vi "MarvinReport.vi"(0 "HEADER1":string="===================================================================\r\n||  Functional and Performance Test  For  DUAL-SERVO- L O W E R  ||\r\n||  P/N  TLM132XX501    S/N:001    Power-Input:18,28,32 +/-0.5V  ||\r\n||  Date:6/12/2007    Time: 15-00  Test-Conductor: Itzik         ||\r\n||  Tester P/N yyyy-yyyyyy-yyyy    S/N:01                        ||\r\n||  POWER SUPPLY P/N xxxxx                                       ||\r\n||  Remarks:                                                     ||\r\n||  You can write here what ever you want                        ||\r\n||                                                               ||\r\n===================================================================", 1 "ATR Or":refnum<vi>, 2 "Steps   pfull":string[][](table)=array602x15[9030 elements] caption="ATR", 3 "Footer UUT":string, 5 "pageNum":i32=13, 6 "InputHeaderArray":string[][](array[string]), 7 "FILE NAME":string="d", 9 "Report Folder":path=path "C:/EPD/ATRS", 11 "Open File":bool caption="Open", 12 "error in (no error)":errorcluster, 13 "REV":string, 14 "Test-Conductor":string) -> (4 "path out":path, 15 "error out":errorcluster)   [LabVIEW 2017]
uses:
  <vilib>/Utility/miscctls.llb/LVRowAndColumnUnsignedTypeDef.ctl
  <vilib>/Utility/NIReport.llb/Append Image to Report (path wrap).vi
  <vilib>/Utility/NIReport.llb/Append Text Table to Report (wrap).vi
  <vilib>/Utility/NIReport.llb/Append Report Text (str wrap).vi
  <vilib>/Utility/NIReport.llb/NI_report.lvclass
  <vilib>/Utility/NIReport.llb/Word/NI_Word.lvclass
  <vilib>/addons/_office/NI_ReportGenerationToolkit.lvlib
panel:
  out "Steps   p31":string[][](table)=[["6.1", "Visual Inspection", "", "", "", "", ""], ["6.1.1", "Verification of Components Not Installed", "N/A", "-", "", "", ""], ["", "", "", "", "", "", ""], ["6.1.2", "Manufacturing Defects", "N/A", "-", "", "", ""], ["", "", "", "", "", "", ""], ["6.2", "Power Supply Testing", "", "", "", "", ""], ["6.2.1", "Input Current Drawn", "", "", "", "", ""], ["6.2.1.1", "DC Input Current", "< 150", "-", "mA", "", ""], ["", "", "", "", "", "", ""], ["6.2.2", "Power Supply Voltages", "", "", "", "", ""], ["6.2.2.1", "12V", "12.0", "+/-0.500", "V", "", ""], ["6.2.2.2", "5V", "5.0", "+/-0.200", "V", "", ""], ["6.2.2.3", "3.3V", "3.3", "+/-0.100", "V", "", ""], ["6.2.2.4", "1.8V", "1.8", "+/-0.100", "V", "", ""], ["", "", "", "", "", "", ""], ["7", "Functional Test Procedure", "", "", "", "", ""], ["7.1", "Weight Check", "4180", "+/-10.00", "gr", "", ""], ["", "", "", "", "", "", ""], ["7.2", "Insulation Resistance Test", "", "", "", "", ""], ["7.2.1", "J3.B to Chassis", "> 1M", "-", "ohms", "", ""], ["7.2.2", "J1.16 to Chassis", "> 100K", "-", "ohms", "", ""], ["", "", "", "", "", "", ""], ["7.2", "Bonding Resistance", "", "", "", "", ""], ["7.2.3", "J1 Body to Chassis", "< 2m", "-", "ohms", "", ""], ["7.2.4", "J2  Body to Chassis", "< 2m", "-", "ohms", "", ""], ["7.2.5", "J3  Body to Chassis", "< 2m", "-", "ohms", "", ""], ["", "", "", "", "", "", ""], ["7.2.1", "CANbus Resistance Test", "", "", "", "", ""], ["7.2.1.1", "J1.17 to J1.18", "> 10K", "-", "ohms", "", ""], ["", "", "", "", "", "", ""], ["7.3", "Sealing Test", "N/A", "-", "", "", ""], ["", "", "", "", "", "", ""], ["7.4", "Communication Test", "", "", "", "", ""], ["7.4.1", "Serial RS-232", "N/A", "-", "", "", ""], ["7.4.2", "CAN Bus", "N/A", "-", "", "", ""], ["", "", "", "", "", "", ""], ["7.5", "Performances Tests", "", "", "", "", ""], ["7.5.1", "Reverse Polarity Test", "", "", "", "", ""], ["7.5.1.1", "DC Input Current", "< 1", "-", "mA", "", ""], ["", "", "", "", "", "", ""], ["7.5.2", "Enable Test", "", "", "", "", ""], ["7.5.2.1", "Fan Speed before Opened Enable ", "6000", "+/-200.0", "rpm", "", ""], ["7.5.2.2", "Fan Speed at Opened Enable ", "0", "+/-200.0", "rpm", "", ""], ["7.5.2.3", "Fan Speed at Closed Enable ", "6000", "+/-200.0", "rpm", "", ""], ["7.5.2.4", "Motor Rotation Direction", "Counter-clockwise (Inlet)", "-", "", "", ""], ["", "", "", "", "", "", ""], ["7.5.3", "Stop Time Test ", "", "", "", "", ""], ["7.5.3.1", "Motor Stop time", "< 50", "-", "sec", "", ""], ["", "", "", "", "", "", ""], ["7.5.4", "Speed Command Test", "", "", "", "", ""], ["7.5.4.1", "Fan Speed", "6000", "+/-200.0", "rpm", "", ""], ["7.5.4.2", "Fan Speed", "11500", "+/-200.0", "rpm", "", ""], ["7.5.4.3", "Fan Speed", "15100", "+/-200.0", "rpm", "", ""], ["", "", "", "", "", "", ""], ["7.5.5", "Temperature Sensor Calibration Test", "", "", "", "", ""], ["7.5.5.1", "Sensor Reading Analog Offset", "0", "+/-0.100", ".", "", ""], ["", "", "", "", "", "", ""], ["7.5.6", "Temperature Control Algorithm Test", "", "", "", "", ""], ["7.5.6.1", "Tair <   68 ± 2 oC", "6000", "+/-200.0", "rpm", "", ""], ["7.5.6.2", "Measured Temp.", "", "", "Deg.", "", ""], ["7.5.6.3", "Tair >= 68 ± 2 oC", "11500", "+/-200.0", "rpm", "", ""], ["7.5.6.4", "Transition Temp.", "", "", "Deg.", "", ""], ["7.5.6.5", "Tair >= 88 ± 2 oC", "15100", "+/-400.0", "rpm", "", ""], ["7.5.6.6", "Transition Temp.", "", "", "Deg.", "", ""], ["7.5.6.7", "Tair <= 80 ± 2 oC", "11500", "+/-200.0", "rpm", "", ""], ["7.5.6.8", "Transition Temp.", "", "", "Deg.", "", ""], ["7.5.6.9", "Tair <= 60 ± 2 oC", "6000", "+/-200.0", "rpm", "", ""], ["7.5.6.10", "Transition Temp.", "", "", "Deg.", "", ""], ["", "", "", "", "", "", ""], ["7.5.7", "Burn-in Test", "", "", "", "", ""], ["7.5.7.1", "DC Input Current", "50", "+/-7.000", "A", "", ""], ["7.5.7.2", "Fan Speed", "15100", "+/-400.0", "rpm", "", ""], ["7.5.7.3", "Ambient Temperature", "25", "+/-13.00", "Deg.", "", ""], ["7.5.7.4", "After 10 min of operation", "", "-", "Deg.", "", ""], ["7.5.7.5", "After 20 min of operation", "", "-", "Deg.", "", ""], ["7.5.7.6", "After 30 min of operation", "", "-", "Deg.", "", ""], ["", "", "", "", "", "", ""], ["8", "Auxiliary", "", "", "", "", ""], ["8.1", "Auxiliary Cooling Fan ON", "60", "+/-2.00", "Deg.", "", ""], ["8.2", "Fan status", "ON", "-", "-", "", ""], ["8.3", "Auxiliary Cooling Fan OFF", "55", "+/-2.00", "Deg.", "", ""], ["8.4", "Fan status", "OFF", "-", "-", "", ""], ["", "", "", "", "", "", ""], ["9", "Motor Temp. Test", "", "", "", "", ""], ["9.1", "60 Degree", "60", "+/-2.00", "Deg.", "", ""], ["9.2", "90 Degree", "90", "+/-2.00", "Deg.", "", ""], ["9.3", "110 Degree", "110", "+/-2.00", "Deg.", "", ""]] caption="ATR"
  out "error out 2":errorcluster
  out "RefArr":u32[](array[numeric])
  in  "Tab Control":T1(tab)=enum."Headers and more"
  out "ERRORS\nLIST":string="<pre>Summery of Results (Fails Only) :   Pos.Cmnd.=0.5V F.B. - FAIL !\t   \nPos.Cmnd.=2.0V F.B. - FAIL !\t       Pos.Cmnd.=4.5V F.B. - FAIL !\t  \nPos.Cmnd.=0.5V F.B  - FAIL !\t       Pos.Cmnd.=2.0V F.B. - FAIL !\t\nPos.Cmnd.=4.5V F.B. - FAIL !\t       Pot. / Pos.Cmnd. 1.5v - FAIL !\t   \nPot./Pos.Cmnd.2.0v  - FAIL !\t       Pot. / Pos.Cmnd. 3.5v - FAIL !\t   \nRelay-->RESET  - FAIL !\t            Relay --> SET - FAIL !\t</pre>"
  out "Steps   p1":string[][](table)=[["Load Firmware - reset", "-", "-", "-", "-", ""], ["Test Communication", "-", "-", "-", "-", ""], ["Set S/N", "-", "-", "-", "-", ""], ["Set Board Number", "-", "-", "-", "-", ""], [" ", "", "", "", "", ""], ["Test Communication", "-", "-", "-", "-", ""], ["Get S/N", "-", "-", "-", "", ""], ["Get Board Number", "-", "-", "-", "", ""], ["Get FW", "-", "-", "-", "", ""], ["Small position command", "", "", "", "", ""], ["Measure delta", "", "", "", "", ""], ["Velocity command", "", "", "", "", ""], ["Velocity command", "", "", "", "", ""], ["Velocity command", "", "", "", "", ""], ["Velocity command", "", "", "", "", ""], ["Velocity command", "", "", "", "", ""]] caption="ATR"
  out "Steps   p2":string[][](table)=[["Load Firmware - reset", "-", "-", "-", "-", ""], ["Test Communication", "-", "-", "-", "-", ""], ["Set S/N", "-", "-", "-", "-", ""], ["Set Board Number", "-", "-", "-", "-", ""], [" ", "", "", "", "", ""], ["Test Communication", "-", "-", "-", "-", ""], ["Get S/N", "-", "-", "-", "", ""], ["Get Board Number", "-", "-", "-", "", ""], ["Get FW", "-", "-", "-", "", ""], ["Small position command", "", "", "", "", ""], ["Measure delta", "", "", "", "", ""], ["Velocity command", "", "", "", "", ""], ["Velocity command", "", "", "", "", ""], ["Velocity command", "", "", "", "", ""], ["Velocity command", "", "", "", "", ""], ["Velocity command", "", "", "", "", ""]] caption="ATR"
  out "Steps   p3":string[][](table)=[["Load Firmware - reset", "-", "-", "-", "-", ""], ["Test Communication", "-", "-", "-", "-", ""], ["Set S/N", "-", "-", "-", "-", ""], ["Set Board Number", "-", "-", "-", "-", ""], [" ", "", "", "", "", ""], ["Test Communication", "-", "-", "-", "-", ""], ["Get S/N", "-", "-", "-", "", ""], ["Get Board Number", "-", "-", "-", "", ""], ["Get FW", "-", "-", "-", "", ""], ["Small position command", "", "", "", "", ""], ["Measure delta", "", "", "", "", ""], ["Velocity command", "", "", "", "", ""], ["Velocity command", "", "", "", "", ""], ["Velocity command", "", "", "", "", ""], ["Velocity command", "", "", "", "", ""], ["Velocity command", "", "", "", "", ""]] caption="ATR"
  in  "Fail  Button":bool
  in  "Pass  Button":bool
  # "e"
  # "e"
  # "<pre>"
  # "for html"
  # "for html"
  # "</pre>"
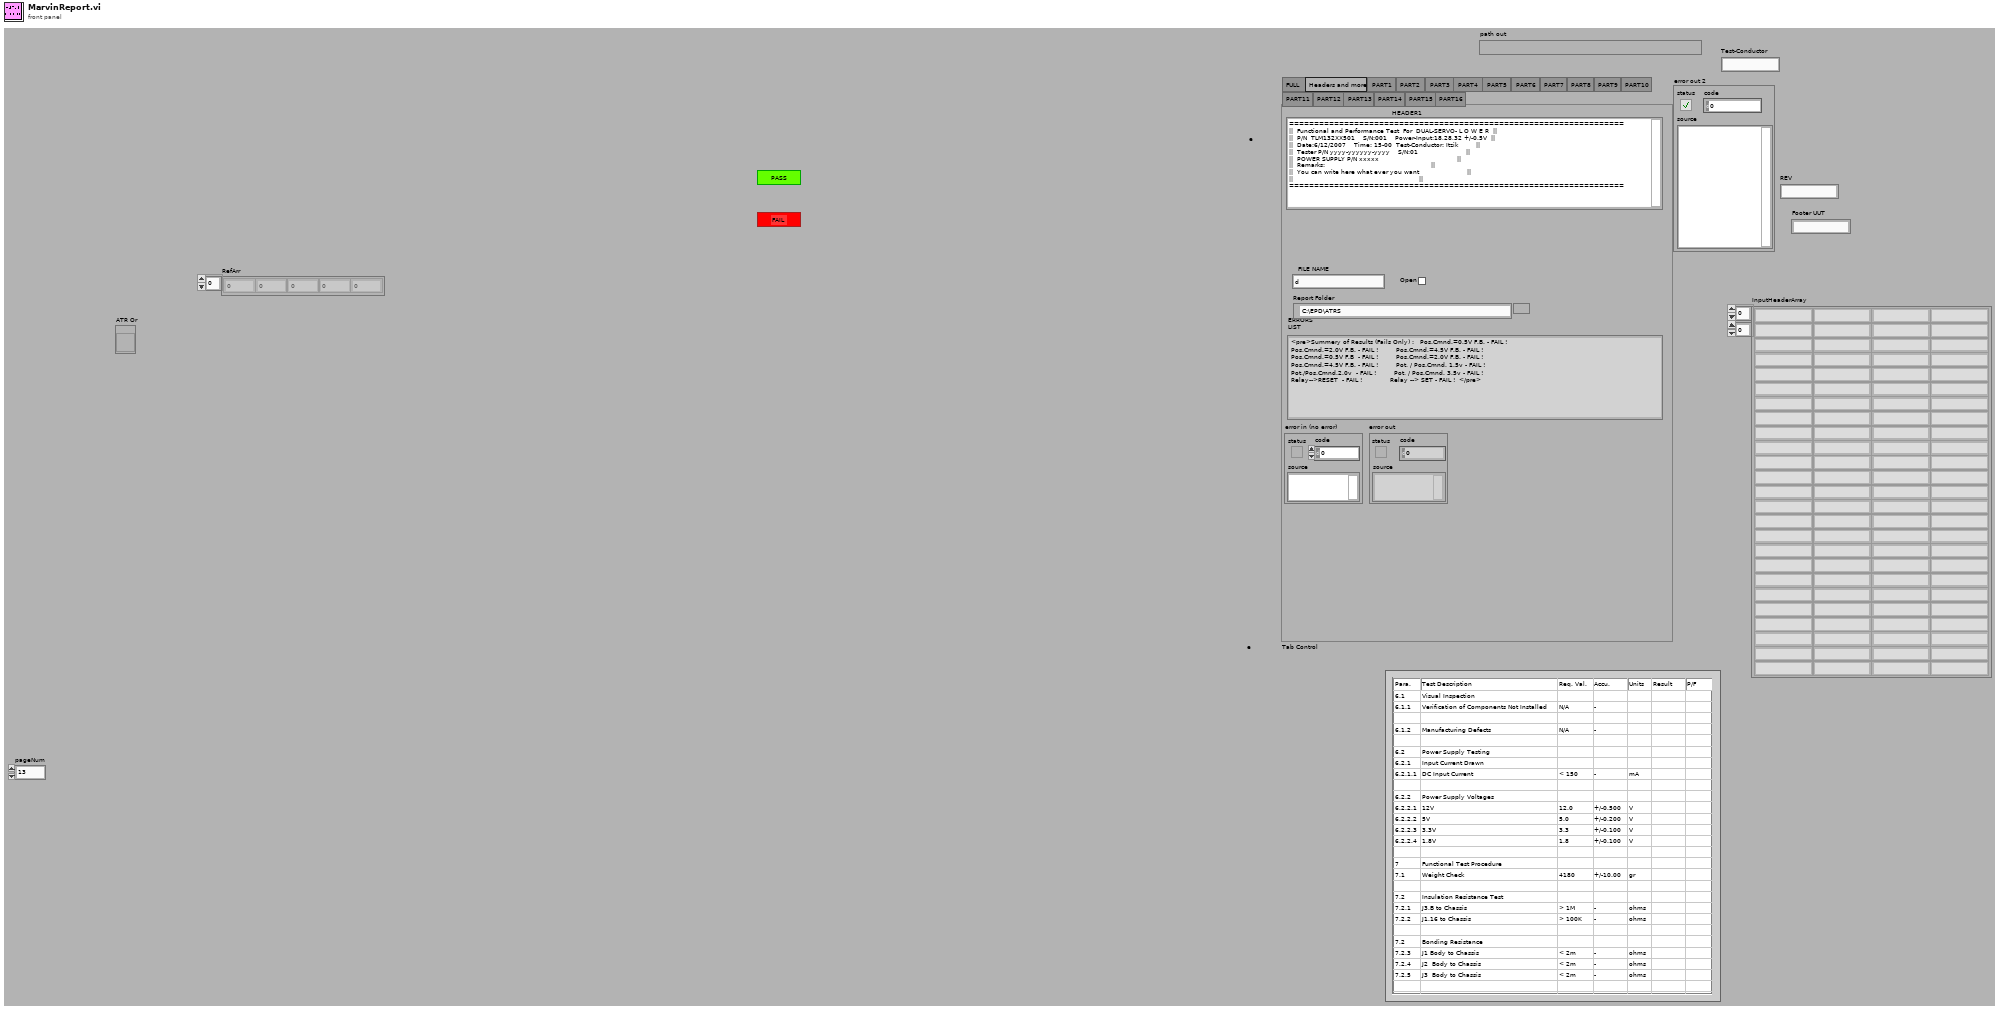
[diagram p1: front panel]
types:
  T1 = enum32{"FULL", "Headers and more", "PART1 ", "PART2 ", "PART3 ", "PART4 ", "PART5 ", "PART6 ", "PART7", "PART8", "PART9", "PART10", "PART11", "PART12", "PART13", "PART14", "PART15", "PART16"}
  T2 = typedef "LVRowAndColumnUnsignedTypeDef.ctl" = cluster{"Row":u32, "Column":u32}
  T3 = cluster{"position (excel)":cluster{"row":i32, "column":i32}, "name (excel)":string, "bookmark (word)":string}
  T4 = cluster{"top":dbl, "left":dbl, "right":dbl, "bottom":dbl}
  T5 = enum16{"Standard Report", "HTML", "Word", "Excel"}
  T6 = cluster{"Italic":enum16{"Italic Unchanged", "Italic On", "Italic Off"}, "Strike Through":enum16{"Strike Through Unchanged", "Strike Through On", "Strike Through Off"}, "Underline":enum16{"Underline Unchanged", "Underline On", "Underline Off"}, "Bold":enum16{"Bold Unchanged", "Bold On", "Bold Off"}}
  T7 = cluster{"charset (-1)":i16, "weight (-1)":i16, "name":string, "size":string}
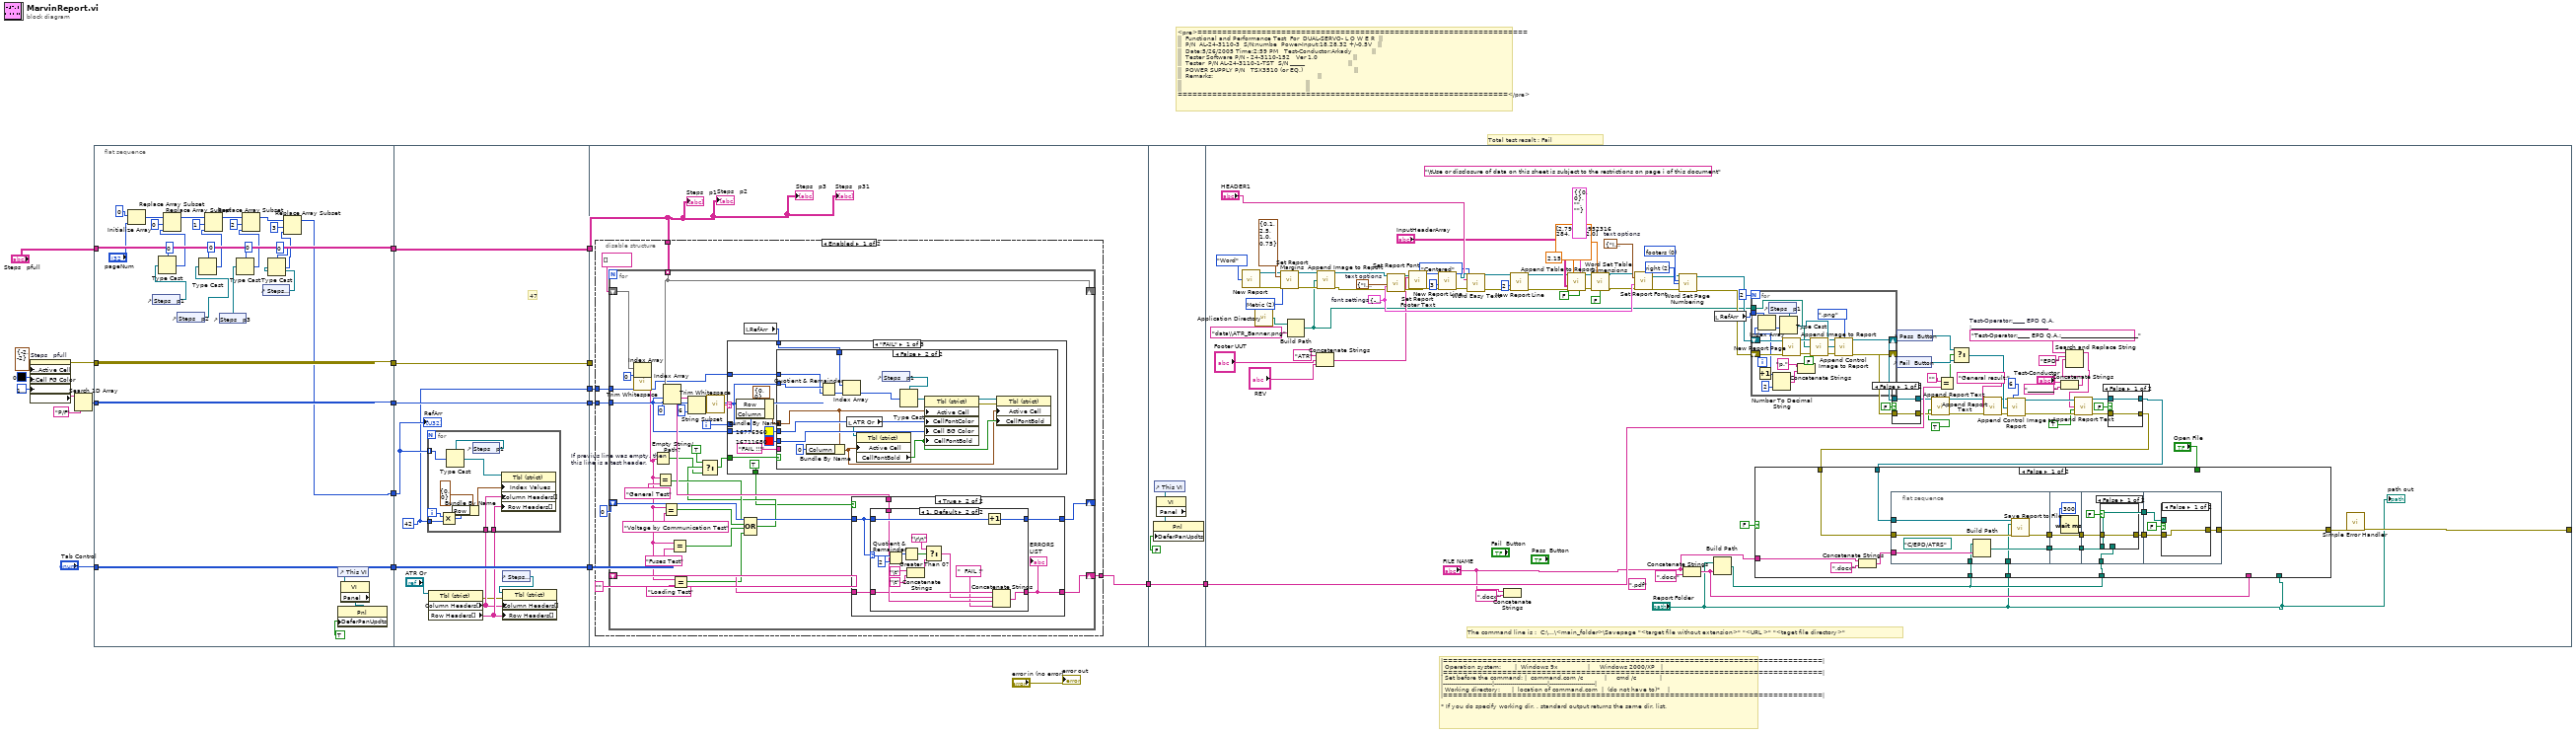
[diagram p0: block diagram]
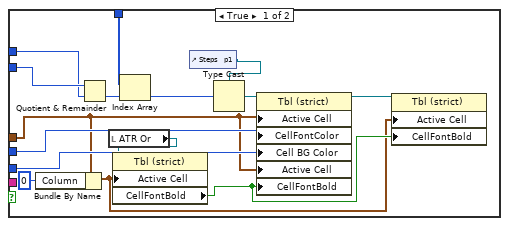
[diagram p2: hidden frame]
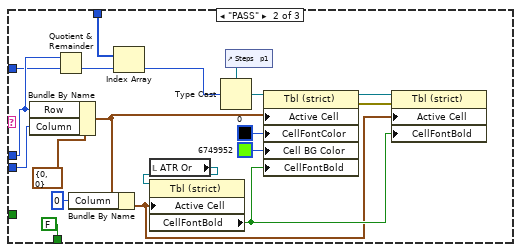
[diagram p3: hidden frame]
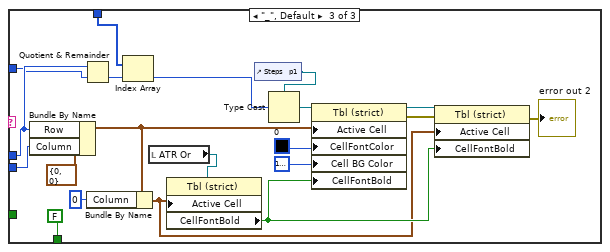
[diagram p4: hidden frame]
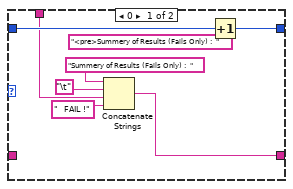
[diagram p6: hidden frame]
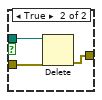
[diagram p9: hidden frame]
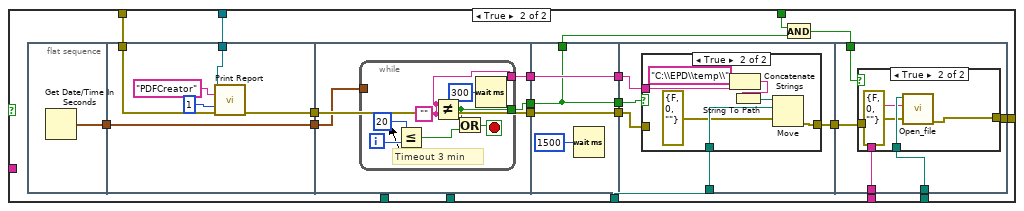
[diagram p10: hidden frame]
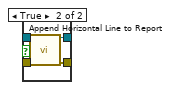
[diagram p13: hidden frame]
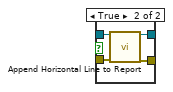
[diagram p14: hidden frame]
diagram:
  # "Total test resalt : Fail"
  # "|=============================================================================|\n| Operation system:       |  Windows 9x               |     Windows 2000/XP   |\n|=============================================================================|\n| Set before the command: |  command.com /c           |     cmd /c            |\n|-------------------------|---------------------------|-----------------------|\n| Working directory:      |  location of command.com  |  (do not have to)*    |\n|=============================================================================|\n\n* If you do specify working dir. , standard output returns the same dir. list."
  # "<pre>===================================================================\n||  Functional and Performance Test  For  DUAL-SERVO- L O W E R  ||\n||  P/N  AL-24-3110-3  S/N:numbe  Power-Input:18,28,32 +/-0.5V   ||\n||  Date:5/26/2005 Time:2:59 PM   Test-Conductor:Arkady          ||\n||  Tester Software P/N - 24-3110-152   Ver 1.0                  ||\n||  Tester  P/N AL-24-3110-1-TST  S/N _____                      ||\n||  POWER SUPPLY P/N   TSX3510 (or EQ.)                          ||\n||  Remarks:                                                     ||\n||                                                               ||\n||                                                               ||\n===================================================================</pre>"
  n1 = property on="Steps   pfull" class="Tbl (strict)"("Active Cell:Active Cell"=cluster{"Row":i32, "Column":i32} {"Row"=-2, "Column"=-2} ("Active Cell"), "Active Cell:Cell FG Color"=u32 0, "Active Cell:Cell Background Color"=u32 16777226) -> (error out=w19:errorcluster, "Column Header Strings[]"=w17:string[])  [unwired: 2 in, 1 out]
  n2 = Search 1D Array(1D array=w17, element="P/F") -> (index of element=w16:i32)  [unwired: 1 in]
  n3 = flat-sequence {
    tunnel: "Tab Control" -> [w49]
    tunnel: w16 -> [w50]
    tunnel: w19 -> [w51]
    tunnel: "Steps   pfull" -> [w52]
    tunnel: [w52] -> w8
    tunnel: [w51] -> w7
    tunnel: [w50] -> w6
    tunnel: [w49] -> w5
    tunnel: [w27] -> w2
    tunnel: [w63] -> w12
    tunnel: [w62] -> w11
    tunnel: [w61] -> w10
    tunnel: [w60] -> w9
    tunnel: w8 -> [w63]
    tunnel: w7 -> [w62]
    tunnel: w6 -> [w61]
    tunnel: w5 -> [w60]
    tunnel: w2 -> [w55]
    tunnel: [w53] -> w1
    tunnel: [w76] -> w4
    tunnel: w12 -> [w74]
    tunnel: w11 -> [_]
    tunnel: w10 -> [w77]
    tunnel: w9 -> [_]
    tunnel: w1 -> [w75]
    tunnel: w4 -> [w230]
    tunnel: [w230] -> w3
    tunnel: [w322] -> _
    tunnel: w3 -> [w309]
    frame #0 {
      n4 = Initialize Array "Initialize Array"(u32 0, "pageNum") -> (w34:u32[])
      n5 = control-ref of="Steps   p1"() -> (w45:refnum<vi>)
      n6 = Type Cast(type=u32 0, x=w45) -> (*(type *) &x=w35:u32)
      n7 = Replace Array Subset(array=w34, new element=w35, index=0) -> (w38:u32[])
      n8 = control-ref of="Steps   p2"() -> (w30:refnum<vi>)
      n9 = Type Cast(type=u32 0, x=w30) -> (*(type *) &x=w39:u32)
      n10 = Replace Array Subset(array=w38, new element=w39, index=1) -> (w44:u32[])
      n11 = control-ref of="Steps   p3"() -> (w24:refnum<vi>)
      n12 = Type Cast(type=u32 0, x=w24) -> (*(type *) &x=w42:u32)
      n13 = Replace Array Subset(array=w44, new element=w42, index=2) -> (w28:u32[])
      n14 = control-ref of="Steps   p31"() -> (w23:refnum<vi>)
      n15 = Type Cast(type=u32 0, x=w23) -> (*(type *) &x=w25:u32)
      n16 = Replace Array Subset(array=w28, new element=w25, index=3) -> (w27:u32[])
      n17 = control-ref of="This VI"() -> (w46:refnum<vi>)
      n18 = property class="VI"(reference=w46) -> ("Panel"=w47:refnum<vi>)  [unwired: 1 in, 2 out]
      n19 = property class="Pnl"(reference=w47, "DeferPanUpdts"=TRUE ("Defer Panel Updates")) -> ()  [unwired: 1 in, 2 out]
    }
    frame #1 {
      w53 = u32 42 ("Row")
      # "47"
      n20 = property class="Tbl (strict)"(reference="ATR Or") -> (error out=w57:errorcluster, "Column Headers[]"=w58:string[], "Row Headers[]"=w59:string[])  [unwired: 1 in, 1 out]
      n21 = for {
        tunnel: w55 -> [w73] mode=indexing
        tunnel: w58 -> [w67]
        tunnel: w59 -> [w66]
        tunnel: w53 -> [w64]
        i -> [w69]
        n22 = Multiply(x=w69, y=w64) -> (x*y=w68:u32)
        n23 = Bundle By Name(cluster=T2 {"Row"=0, "Column"=0} ("Index Values"), "Row"=w68) -> (w70:T2)
        n24 = control-ref of="Steps   p1"() -> (w65:refnum<vi>)
        n25 = Type Cast(type=w65, x=w73) -> (*(type *) &x=w72:refnum<vi>)
        n26 = property class="Tbl (strict)"(reference=w72, "Index Values"=w70, "Column Headers[]"=w67, "Row Headers[]"=w66) -> ()  [unwired: 1 in, 2 out]
      }
      n27 = control-ref of="Steps   pfull"() -> (w54:refnum<vi>)
      n28 = property class="Tbl (strict)"(reference=w54, error in=w57, "Column Headers[]"=w58, "Row Headers[]"=w59) -> ()  [unwired: 2 out]
      "RefArr" <- w55
    }
    frame #2 {
      n29 = disable-structure shown="Enabled" {
        disable-tunnel: w77 -> [w84 _]
        disable-tunnel: [w83 _] -> w76
        disable-tunnel: w74 -> [w79 _]
        disable-tunnel: w75 -> [w78 _]
        frame Enabled {
          n30 = for {
            tunnel: w79 -> [w114] mode=indexing
            shift-right: [w114] -> _
            shift-left: string[] [] ("ATR in") -> [w113]
            tunnel: w84 -> [w90]
            shift-right: [w105] -> w83
            shift-left: "" ("trimmed string") -> [w109]
            shift-right: [w108] -> _
            shift-left: 0 -> [w107]
            tunnel: w78 -> [w85]
            i -> [w91]
            n31 = Index Array(array=w113, index=0) -> (element=w111:string)
            n32 = call <vilib>:"Trim Whitespace.vi"("string"=w111) -> ("trimmed string"=w86:string)  [unwired: 1 in]
            n33 = Empty String/Path? "If previus line was empty, then\nthis line is a test header."(string/path=w86) -> (empty?=w93:bool)
            n34 = Equal?(x=w86, y="General Test") -> (x = y?=w102:bool)
            n35 = Equal?(x=w86, y="Voltage by Communication Test") -> (x = y?=w97:bool)
            n36 = Index Array(array=w114, index #1=w90, index #2=0) -> (element #1=w110:string, element #2=w106:string)
            n37 = Equal?(x=w86, y="Fuses Test") -> (x = y?=w98:bool)
            n38 = Equal?(x=w86, y="Loading Test") -> (x = y?=w99:bool)
            n39 = String Subset(string=w110, length (rest)=6 ("length (rest)")) -> (substring=w115:string)  [unwired: 1 in]
            n40 = call <vilib>:"Trim Whitespace.vi"("string"=w115) -> ("trimmed string"=w92:string)  [unwired: 1 in]
            n41 = local read "RefArr"() -> (w87:u32[])
            n42 = Compound Arithmetic op=OR(w102, w97, w98, w99) -> (w100:bool)
            n43 = Select(t=TRUE, s=w100, f=w93) -> (s? t:f=w89:bool)
            n44 = case shown="\"FAIL\"" w92 {
              tunnel: w91 -> [w119 w172 w193]
              tunnel: w90 -> [w121 w176 w196]
              tunnel: w89 -> [w123 _ _]
              tunnel: [TRUE FALSE FALSE] -> w88
              tunnel: w87 -> [w120 w170 w192]
              tunnel: w85 -> [w117 w159 w178]
              frame "FAIL" {
                n45 = Bundle By Name(cluster=cluster{"Row":i32, "Column":i32} {"Row"=0, "Column"=0} ("Active Cell"), "Row"=w119, "Column"=w121) -> (w127:cluster{"Row":i32, "Column":i32})
                n46 = case shown="False" w123 {
                  tunnel: w127 -> [w135 w147]
                  tunnel: u32 16776960 -> [w142 w158]
                  tunnel: u32 16711680 -> [w141 w157]
                  tunnel: "FAIL !!!" ("string") -> [_ _]
                  tunnel: w120 -> [w139 w154]
                  tunnel: w119 -> [w138 w155]
                  tunnel: w117 -> [w128 w143]
                  frame True {
                    n47 = Bundle By Name(cluster=w135, "Column"=0) -> (w131:cluster{"Row":i32, "Column":i32})
                    n48 = Quotient & Remainder(x=w138, y=w128) -> (floor(x/y)=w140:u32)  [unwired: 1 out]
                    n49 = local read "ATR Or"() -> (w129:refnum<vi>)
                    n50 = property class="Tbl (strict)"(reference=w129, "Active Cell"=w131) -> ("CellFontBold"=w132:bool)  [unwired: 1 in, 2 out]
                    n51 = Index Array(array=w139, index=w140) -> (element=w136:u32)
                    n52 = control-ref of="Steps   p1"() -> (w130:refnum<vi>)
                    n53 = Type Cast(type=w130, x=w136) -> (*(type *) &x=w137:refnum<vi>)
                    n54 = property class="Tbl (strict)"(reference=w137, "Active Cell"=w135, "CellFontColor"=w142, "Cell BG Color"=w141, "Active Cell"=w135, "CellFontBold"=w132) -> (reference out=w133:refnum<vi>)  [unwired: 1 in, 1 out]
                    n55 = property class="Tbl (strict)"(reference=w133, "Active Cell"=w131, "CellFontBold"=w132) -> ()  [unwired: 1 in, 2 out]
                  }
                  frame False {
                    n56 = Bundle By Name(cluster=w147, "Column"=0) -> (w146:cluster{"Row":i32, "Column":i32})
                    n57 = Quotient & Remainder(x=w155, y=w143) -> (floor(x/y)=w156:u32)  [unwired: 1 out]
                    n58 = Index Array(array=w154, index=w156) -> (element=w153:u32)
                    n59 = local read "ATR Or"() -> (w145:refnum<vi>)
                    n60 = property class="Tbl (strict)"(reference=w145, "Active Cell"=w146) -> ("CellFontBold"=w149:bool)  [unwired: 1 in, 2 out]
                    n61 = control-ref of="Steps   p1"() -> (w144:refnum<vi>)
                    n62 = Type Cast(type=w144, x=w153) -> (*(type *) &x=w152:refnum<vi>)
                    n63 = property class="Tbl (strict)"(reference=w152, "Active Cell"=w147, "CellFontColor"=w158, "Cell BG Color"=w157, "CellFontBold"=w149) -> (reference out=w151:refnum<vi>, error out=w150:errorcluster)  [unwired: 1 in]
                    n64 = property class="Tbl (strict)"(reference=w151, error in=w150, "Active Cell"=w146, "CellFontBold"=w149) -> ()  [unwired: 2 out]
                  }
                }
              }
              frame "PASS" {
                n65 = Bundle By Name(cluster=cluster{"Row":i32, "Column":i32} {"Row"=0, "Column"=0} ("Active Cell"), "Row"=w172, "Column"=w176) -> (w163:cluster{"Row":i32, "Column":i32})
                n66 = Quotient & Remainder(x=w172, y=w159) -> (floor(x/y)=w171:u32)  [unwired: 1 out]
                n67 = Bundle By Name(cluster=w163, "Column"=0) -> (w162:cluster{"Row":i32, "Column":i32})
                n68 = Index Array(array=w170, index=w171) -> (element=w169:u32)
                n69 = local read "ATR Or"() -> (w160:refnum<vi>)
                n70 = property class="Tbl (strict)"(reference=w160, "Active Cell"=w162) -> ("CellFontBold"=w165:bool)  [unwired: 1 in, 2 out]
                n71 = control-ref of="Steps   p1"() -> (w161:refnum<vi>)
                n72 = Type Cast(type=w161, x=w169) -> (*(type *) &x=w168:refnum<vi>)
                n73 = property class="Tbl (strict)"(reference=w168, "Active Cell"=w163, "CellFontColor"=u32 0, "Cell BG Color"=u32 6749952, "CellFontBold"=w165) -> (reference out=w166:refnum<vi>, error out=w167:errorcluster)  [unwired: 1 in]
                n74 = property class="Tbl (strict)"(reference=w166, error in=w167, "Active Cell"=w162, "CellFontBold"=w165) -> ()  [unwired: 2 out]
              }
              frame "_", Default {
                n75 = Bundle By Name(cluster=cluster{"Row":i32, "Column":i32} {"Row"=0, "Column"=0} ("Active Cell"), "Row"=w193, "Column"=w196) -> (w186:cluster{"Row":i32, "Column":i32})
                n76 = Quotient & Remainder(x=w193, y=w178) -> (floor(x/y)=w194:u32)  [unwired: 1 out]
                n77 = Bundle By Name(cluster=w186, "Column"=0) -> (w182:cluster{"Row":i32, "Column":i32})
                n78 = Index Array(array=w192, index=w194) -> (element=w191:u32)
                n79 = local read "ATR Or"() -> (w180:refnum<vi>)
                n80 = property class="Tbl (strict)"(reference=w180, "Active Cell"=w182) -> ("CellFontBold"=w183:bool)  [unwired: 1 in, 2 out]
                n81 = control-ref of="Steps   p1"() -> (w181:refnum<vi>)
                n82 = Type Cast(type=w181, x=w191) -> (*(type *) &x=w188:refnum<vi>)
                n83 = property class="Tbl (strict)"(reference=w188, "Active Cell"=w186, "CellFontColor"=u32 0, "Cell BG Color"=u32 16777226, "CellFontBold"=w183) -> (reference out=w185:refnum<vi>, error out=w184:errorcluster)  [unwired: 1 in]
                n84 = property class="Tbl (strict)"(reference=w185, error in=w184, "Active Cell"=w182, "CellFontBold"=w183) -> (error out=→"error out 2":errorcluster)  [unwired: 1 out]
              }
            }
            n85 = case shown="True" w88 {
              tunnel: w109 -> [w199 w201]
              tunnel: [w199 w200] -> w105
              tunnel: w107 -> [w198 w203]
              tunnel: [w198 w204] -> w108
              tunnel: w106 -> [_ w202]
              frame False {
              }
              frame True {
                n86 = case shown="1, Default" w203 {
                  selector: w203 -> [_ w225]
                  tunnel: [w206 w215] -> w204
                  tunnel: w203 -> [w211 w226]
                  tunnel: w202 -> [w210 w222]
                  tunnel: [w208 w221] -> w200
                  tunnel: w201 -> [_ w220]
                  frame 0 {
                    (unwired) "<pre>Summery of Results (Fails Only) :  "
                    n87 = Concatenate Strings("Summery of Results (Fails Only) :  ", "\t", w210, "  FAIL !" ("string")) -> (w208:string)
                    n88 = Increment(x=w211) -> (x+1=w206:i32)
                  }
                  frame 1, Default {
                    n89 = Quotient & Remainder(x=w225, y=2) -> (x-y*floor(x/y)=w223:i32)  [unwired: 1 out]
                    n90 = Greater Than 0?(x=w223) -> (x > 0?=w219:bool)
                    n91 = Concatenate Strings("\t", "\t") -> (w214:string)
                    n92 = Select(t="\r\n", s=w219, f=w214) -> (s? t:f=w217:string)
                    n93 = Increment(x=w226) -> (x+1=w215:i32)
                    n94 = Concatenate Strings(w220, w217, w222, "  FAIL !" ("string")) -> (w221:string)
                  }
                }
                "ERRORS\nLIST" <- w200
              }
            }
          }
        }
        frame Disabled {
        }
      }
      "Steps   p1" <- w74
      "Steps   p2" <- w74
      "Steps   p31" <- w74
      "Steps   p3" <- w74
    }
    frame #3 {
      n95 = control-ref of="This VI"() -> (w227:refnum<vi>)
      n96 = property class="VI"(reference=w227) -> ("Panel"=w228:refnum<vi>)  [unwired: 1 in, 2 out]
      n97 = property class="Pnl"(reference=w228, "DeferPanUpdts"=FALSE ("Defer Panel Updates")) -> ()  [unwired: 1 in, 2 out]
    }
    frame #4 {
      w265 = u16 2 items=["Default", "US", "Metric"] ("measurement system (default)")
      (unwired) "\tUse or disclosure of data on this sheet is subject to the restrictions on page i of this document" ("center footer text")
      w276 = u16 2 items=["left", "center", "right"] ("alignment (right)")
      w277 = u16 0 items=["footers", "headers"] ("position (footers)")
      (unwired) ".pdf" ("File Name")
      w310 = T6 {"Italic"=enum."Italic Off", "Strike Through"=enum."Strike Through Off", "Underline"=enum."Underline Off", "Bold"=enum."Bold Off"}  # text options
      w323 = T6 {"Italic"=enum."Italic Off", "Strike Through"=enum."Strike Through Off", "Underline"=enum."Underline Off", "Bold"=enum."Bold Off"}  # text options
      w305 = "Test-Operator:____ EPD Q.A.:__________________________"  # Test-Operator:____ EPD Q.A.:__________________________
      w311 = T7 {"charset (-1)"=-1, "weight (-1)"=-1, "name"="Tahoma", "size"="12"}  # font settings
      # "The command line is :  C:\\...\\<main_folder>\\Savepage \"<target file without extension>\" \"<URL >\" \"<taget file directory>\""
      n98 = call <vilib>:"New Report.vi"("report type"=T5."Word") -> ("report out"=w263:refnum<class "NI_report.lvclass">, "error out"=w264:errorcluster)  [unwired: 13 in]
      n99 = call <vilib>:"Application Directory.vi"() -> ("Application Directory"=w258:path)
      n100 = call-dynamic "Set Report Margins.vi"("report in"=w263, "margins (1.00)"=T4 {"top"=0.1, "left"=2.5, "right"=1.0, "bottom"=0.75}, "measurement system (default)"=w265, "error in (no error)"=w264) -> ("report out"=w262:refnum<class "NI_report.lvclass">, "error out"=w261:errorcluster)  [unwired: 9 in, 1 out]
      n101 = Build Path(base path=w258, name or relative path="data\\ATR_Banner.png") -> (appended path=w256:path)
      n102 = Concatenate Strings("ATR" ("string"), "Footer UUT", "REV") -> (w268:string)
      n103 = call-poly <vilib>:"Append Image to Report.vi"("report in"=w262, "path or URL of image"=w256, "error in (no error)"=w261) -> ("report out"=w259:refnum<class "NI_report.lvclass">, "error out"=w260:errorcluster)  [unwired: 9 in, 2 out]
      n104 = call-dynamic "Set Report Font.vi"("report in"=w259, "text options"=w323, "font settings"=w311, "error in (no error)"=w260) -> ("report out"=w296:refnum<class "NI_report.lvclass">, "error out"=w293:errorcluster)  [unwired: 9 in, 1 out]
      n105 = call-dynamic "Set Report Footer Text.vi"("report in"=w296, "left footer text"=w268, "error in (no error)"=w293) -> ("report out"=w295:refnum<class "NI_report.lvclass">, "error out"=w294:errorcluster)  [unwired: 11 in]
      n106 = call-dynamic "New Report Line.vi"("report in"=w295, "number of lines (1)"=3, "error in (no error)"=w294) -> ("report out"=w249:refnum<class "NI_report.lvclass">, "error out"=w248:errorcluster)  [unwired: 11 in]
      n107 = call <vilib>:"Word Easy Text.vi"("report in"=w249, "text"="HEADER1", "alignment (left)"=enum16{"Left", "Centered", "Right", "Justify"}."Centered", "error in (no error)"=w248) -> ("report out"=w234:refnum<class "NI_report.lvclass">, "error out"=w235:errorcluster)  [unwired: 9 in, 1 out]
      n108 = Concatenate Strings("FILE NAME", ".docx" ("File Name")) -> ()  [unwired: 1 out]
      n109 = call-dynamic "New Report Line.vi"("report in"=w234, "number of lines (1)"=2, "error in (no error)"=w235) -> ("report out"=w233:refnum<class "NI_report.lvclass">, "error out"=w232:errorcluster)  [unwired: 11 in]
      n110 = call-poly <vilib>:"Append Table to Report.vi"("report in"=w233, "column width (1)"=2.15, "MS Office parameters"=T3 {"position (excel)"={"row"=0, "column"=0}, "name (excel)"="", "bookmark (word)"=""}, "text data"="InputHeaderArray", "error in (no error)"=w232, "show grid lines (YES)"=FALSE) -> ("report out"=w240:refnum<class "NI_report.lvclass">, "error out"=w239:errorcluster)  [unwired: 6 in, 2 out]
      n111 = call <vilib>:"Word Set Table Dimensions.vi"("report in"=w240, "table column widths"=sgl[] [2.8, 2.0, 2.0], "error in (no error)"=w239, "fit to page width? (F)"=FALSE) -> ("report out"=w242:refnum<class "NI_report.lvclass">, "error out"=w243:errorcluster)  [unwired: 10 in]
      n112 = call-dynamic "Set Report Font.vi"("report in"=w242, "text options"=w310, "font settings"=w311, "error in (no error)"=w243) -> ("report out"=w253:refnum<class "NI_report.lvclass">, "error out"=w252:errorcluster)  [unwired: 9 in, 1 out]
      n113 = call <vilib>:"Word Set Page Numbering.vi"("report in"=w253, "position (footers)"=w277, "alignment (right)"=w276, "error in (no error)"=w252) -> ("report out"=w279:refnum<class "NI_report.lvclass">, "error out"=w278:errorcluster)  [unwired: 10 in]
      n114 = Concatenate Strings("FILE NAME", ".docx" ("File Name")) -> (w282:string)
      n115 = Build Path(base path="Report Folder", name or relative path=w282) -> (appended path=w273:path)
      n116 = local read "RefArr"() -> (w274:u32[])
      n117 = for {
        N: 2 -> [_]
        tunnel: w274 -> [w435]
        shift-right: [w440] -> w288
        shift-left: w278 -> [w441]
        shift-right: [w439] -> w287
        shift-left: w279 -> [w442]
        tunnel: w256 -> [w428]
        i -> [w433]
        (unwired) FALSE ("append on new line? (F)")
        n118 = Increment(x=w433) -> (x+1=w445:i32)
        n119 = Index Array(array=w435, index=w433) -> (element=w434:u32)
        n120 = control-ref of="Steps   p1"() -> (w437:refnum<vi>)
        n121 = Number To Decimal String(number=w445, width (-)=i16 2) -> (decimal integer string=w443:string)
        n122 = Type Cast(type=w437, x=w434) -> (*(type *) &x=w438:refnum<vi>)
        n123 = call-dynamic "New Report Page.vi"("report in"=w442, "error in (no error)"=w441) -> ("report out"=w431:refnum<class "NI_report.lvclass">, "error out"=w432:errorcluster)  [unwired: 12 in]
        n124 = Concatenate Strings("p.", w443) -> ()  [unwired: 1 out]
        n125 = call-poly <vilib>:"Append Image to Report.vi"("report in"=w431, "path or URL of image"=w428, "error in (no error)"=w432) -> ("report out"=w430:refnum<class "NI_report.lvclass">, "error out"=w429:errorcluster)  [unwired: 9 in, 2 out]
        n126 = call-dynamic "Append Control Image to Report.vi"("report in"=w430, "image file type (.jpg)"=enum16{".jpg", ".png"}.".png" ("image file type(.jpg)"), "ctrl reference"=w438, "error in (no error)"=w429) -> ("report out"=w439:refnum<class "NI_report.lvclass">, "error out"=w440:errorcluster)  [unwired: 8 in, 2 out]
      }
      n127 = case shown="False" FALSE {
        tunnel: [w447 w452] -> w308
        tunnel: [w448 w451] -> w307
        tunnel: w288 -> [w447 w450]
        tunnel: w287 -> [w448 w449]
        frame False {
        }
        frame True {
          n128 = call-dynamic "Append Horizontal Line to Report.vi"("report in"=w449, "error in (no error)"=w450) -> ("report out"=w451:refnum<class "NI_report.lvclass">, "error out"=w452:errorcluster)  [unwired: 12 in]
        }
      }
      n129 = control-ref of="Fail  Button"() -> (w318:refnum<vi>)
      n130 = control-ref of="Pass  Button"() -> (w319:refnum<vi>)
      n131 = call-poly <vilib>:"Append Report Text.vi"("report in"=w307, "append on new line? (F)"=TRUE, "error in (no error)"=w308) -> ("report out"=w251:refnum<class "NI_report.lvclass">, "error out"=w250:errorcluster)  [unwired: 9 in, 2 out]
      n132 = Equal?(x="", y=w309) -> (x = y?=w316:bool)
      n133 = Select(t=w319, s=w316, f=w318) -> (s? t:f=w320:refnum<vi>)
      n134 = call-poly <vilib>:"Append Report Text.vi"("report in"=w251, "text"="General result:", "error in (no error)"=w250) -> ("report out"=w314:refnum<class "NI_report.lvclass">, "error out"=w315:errorcluster)  [unwired: 9 in, 2 out]
      n135 = call-dynamic "Append Control Image to Report.vi"("report in"=w314, "alignment (default)"=6, "ctrl reference"=w320, "error in (no error)"=w315) -> ("report out"=w312:refnum<class "NI_report.lvclass">, "error out"=w313:errorcluster)  [unwired: 8 in, 2 out]
      n136 = Concatenate Strings("Test-Conductor", "_________") -> (w300:string)
      n137 = Search and Replace String(input string=w305, search string="EPD", replace string=w300) -> (result string=w302:string)  [unwired: 5 in, 3 out]
      n138 = call-poly <vilib>:"Append Report Text.vi"("report in"=w312, "text"=w302, "append on new line? (F)"=TRUE, "error in (no error)"=w313) -> ("report out"=w298:refnum<class "NI_report.lvclass">, "error out"=w297:errorcluster)  [unwired: 8 in, 2 out]
      n139 = case shown="False" FALSE {
        tunnel: w298 -> [w454 w458]
        tunnel: w297 -> [w453 w457]
        tunnel: [w453 w456] -> w286
        tunnel: [w454 w455] -> w284
        frame False {
        }
        frame True {
          n140 = call-dynamic "Append Horizontal Line to Report.vi"("report in"=w458, "error in (no error)"=w457) -> ("report out"=w455:refnum<class "NI_report.lvclass">, "error out"=w456:errorcluster)  [unwired: 12 in]
        }
      }
      n141 = case shown="False" FALSE {
        tunnel: [w334 w372] -> w281
        tunnel: w286 -> [w338 w371]
        tunnel: w273 -> [w330 w370]
        tunnel: w282 -> [_ w369]
        tunnel: "Report Folder" -> [_ w368]
        tunnel: w284 -> [w337 w367]
        tunnel: "Open File" -> [_ w365]
        tunnel: "FILE NAME" -> [w328 _]
        tunnel: w273 -> [w325 _]
        tunnel: "Report Folder" -> [w324 _]
        frame False {
          n142 = Concatenate Strings(w328, ".docx" ("File Name")) -> (w326:string)
          n143 = flat-sequence {
            tunnel: w338 -> [w345]
            tunnel: w337 -> [w343]
            tunnel: [w344] -> w336
            tunnel: [w342] -> w333
            tunnel: w326 -> [w341]
            tunnel: w325 -> [w340]
            tunnel: w324 -> [w339]
            tunnel: w336 -> [w348]
            tunnel: [w348] -> w335
            tunnel: w333 -> [w346]
            tunnel: [w346] -> w332
            tunnel: w335 -> [w353]
            tunnel: w332 -> [w351]
            tunnel: [w349] -> w331
            tunnel: w330 -> [w352]
            tunnel: [w351] -> w329
            tunnel: [w358] -> w334
            tunnel: w331 -> [w359]
            tunnel: w329 -> [w357]
            frame #0 {
              (unwired) path "C:/EPD/ATRS" ("report file path")
              n144 = Build Path(base path=w340, name or relative path=w341) -> (appended path=w342:path)
              n145 = call-dynamic "Save Report to File.vi"("report in"=w343, "report file path"=w339, "error in (no error)"=w345) -> ("error out"=w344:errorcluster)  [unwired: 11 in, 1 out]
            }
            frame #1 {
              n146 = Wait (ms)(milliseconds to wait=u32 300) -> ()  [unwired: 1 out]
            }
            frame #2 {
              n147 = case shown="False" FALSE {
                tunnel: w353 -> [w354 w355]
                tunnel: w352 -> [_ _]
                tunnel: w351 -> [_ _]
                tunnel: [w354 w355] -> w349
                frame False {
                }
                frame True {
                }
              }
            }
            frame #3 {
              n148 = case shown="False" FALSE {
                tunnel: w359 -> [w360 w363]
                tunnel: [w360 w362] -> w358
                tunnel: w357 -> [_ w361]
                frame False {
                }
                frame True {
                  n149 = Delete(path (use dialog)=w361, error in=w363) -> (error out=w362:errorcluster)  [unwired: 3 in, 2 out]
                }
              }
            }
          }
        }
        frame True {
          n150 = flat-sequence {
            tunnel: [w383] -> w382
            tunnel: w367 -> [w387]
            tunnel: w371 -> [w386]
            tunnel: [w385] -> w381
            tunnel: [w384] -> w380
            tunnel: w382 -> [w384]
            tunnel: w381 -> [w393]
            tunnel: w380 -> [w392]
            tunnel: [w393] -> w379
            tunnel: [w391] -> w378
            tunnel: [w390] -> w377
            tunnel: w379 -> [w404]
            tunnel: w378 -> [w403]
            tunnel: w377 -> [w401]
            tunnel: [w404] -> w376
            tunnel: [w403] -> w375
            tunnel: [w401] -> w364
            tunnel: [w401] -> w374
            tunnel: w376 -> [w409]
            tunnel: w375 -> [w408]
            tunnel: w374 -> [w407]
            tunnel: w370 -> [w406]
            tunnel: [w405] -> w373
            tunnel: w373 -> [w422]
            tunnel: w368 -> [w421]
            tunnel: w369 -> [w420]
            tunnel: [w419] -> w372
            tunnel: w366 -> [w418]
            frame #0 {
              n151 = Get Date/Time In Seconds() -> (seconds since 1Jan1904=w383:timestamp)
            }
            frame #1 {
              n152 = call-dynamic "Print Report.vi"("report in"=w387, "printer name (default)"="PDFCreator", "number of copies (1)"=1, "error in (no error)"=w386) -> ("error out"=w385:errorcluster)  [unwired: 10 in, 1 out]
            }
            frame #2 {
              n153 = while {
                tunnel: w392 -> [_]
                tunnel: [w394] -> w391
                tunnel: [w395] -> w390
                i -> [w398]
                stop <- w399 stop-if-true
                w394 = ""
                # "Timeout 3 min"
                n154 = Less Or Equal?(x=20, y=w398) -> (x <= y?=w396:bool)
                n155 = Not Equal?(x=w394, y=w394) -> (x != y?=w395:bool)
                n156 = Or(x=w395, y=w396) -> (x .or. y?=w399:bool)
                n157 = Wait (ms)(milliseconds to wait=u32 300) -> ()  [unwired: 1 out]
              }
            }
            frame #3 {
              n158 = Wait (ms)(milliseconds to wait=u32 1500) -> ()  [unwired: 1 out]
            }
            frame #4 {
              n159 = case shown="True" w407 {
                tunnel: w409 -> [w410 _]
                tunnel: [w410 w417] -> w405
                tunnel: w408 -> [_ w415]
                tunnel: w406 -> [_ w412]
                frame False {
                }
                frame True {
                  n160 = Concatenate Strings("C:\\EPD\\temp\\", w415) -> (w414:string)
                  n161 = String To Path(string=w414) -> (path=w413:path)
                  n162 = Move(source path=w413, error in=errorcluster {"status"=FALSE, "code"=0, "source"=""}, 10:w412) -> (error out=w417:errorcluster)  [unwired: 2 in, 2 out]
                }
              }
            }
            frame #5 {
              n163 = case shown="True" w418 {
                tunnel: w422 -> [w423 _]
                tunnel: [w423 w427] -> w419
                tunnel: w421 -> [_ w426]
                tunnel: w420 -> [_ w425]
                frame False {
                }
                frame True {
                  n164 = call "Open_file.vi"("error in"=errorcluster {"status"=FALSE, "code"=0, "source"=""}, "File Name input"=w425, "Work-Place path\n(with the webarch.exe)"=w426) -> ("error out"=w427:errorcluster)  [unwired: 6 in]
                }
              }
            }
          }
          n165 = And(x=w365, y=w364) -> (x .and. y?=w366:bool)
        }
      }
      n166 = call <vilib>:"Simple Error Handler.vi"("error in (no error)"=w281) -> ("error out"=w322:errorcluster)  [unwired: 4 in, 4 out]
      "path out" <- "Report Folder"
    }
  }
  "error out" <- "error in (no error)"
